vi "Calculate Response.vi"(0 "Neural Network In":T1={"Weigths"=[], "Last Layer Linear"=TRUE, "Add Bias Inputs"=TRUE, "# Inputs"=0, "# Output Neurons/Outputs"=0, "Inputs Scaling"={"X Scaling Vector"=[], "Y Scaling Vector"=[]}, "Outputs Scaling"={"X Scaling Vector"=[], "Y Scaling Vector"=[]}}, 5 "Inputs":dbl[](array[numeric]), 11 "Error In":errorcluster) -> (4 "Neural Network Out":T1={"Weigths"=[], "Last Layer Linear"=TRUE, "Add Bias Inputs"=TRUE, "# Inputs"=0, "# Output Neurons/Outputs"=0, "Inputs Scaling"={"X Scaling Vector"=[], "Y Scaling Vector"=[]}, "Outputs Scaling"={"X Scaling Vector"=[], "Y Scaling Vector"=[]}}, 6 "Outputs":dbl[](array[numeric]), 15 "Error Out":errorcluster)   [LabVIEW 2013, in "Super Simple Neural Network.lvlib"]
doc: "This VI calculates the output values of the network based on the input values. \n\nThis VI also uses the scaling information generated by the teaching algorithm to scale the inputs and outputs of the network. This means that you can work with any values as long as you have tought the network in that specific range."
uses:
  Super Simple Neural Network.lvlib
  Types/Neural Network.ctl
  Types/2D Array.ctl
  Types/Scaling Info.ctl
  <vilib>/Analysis/baseanly.llb/A x Vector.vi
  <vilib>/Analysis/NI_AALBase.lvlib
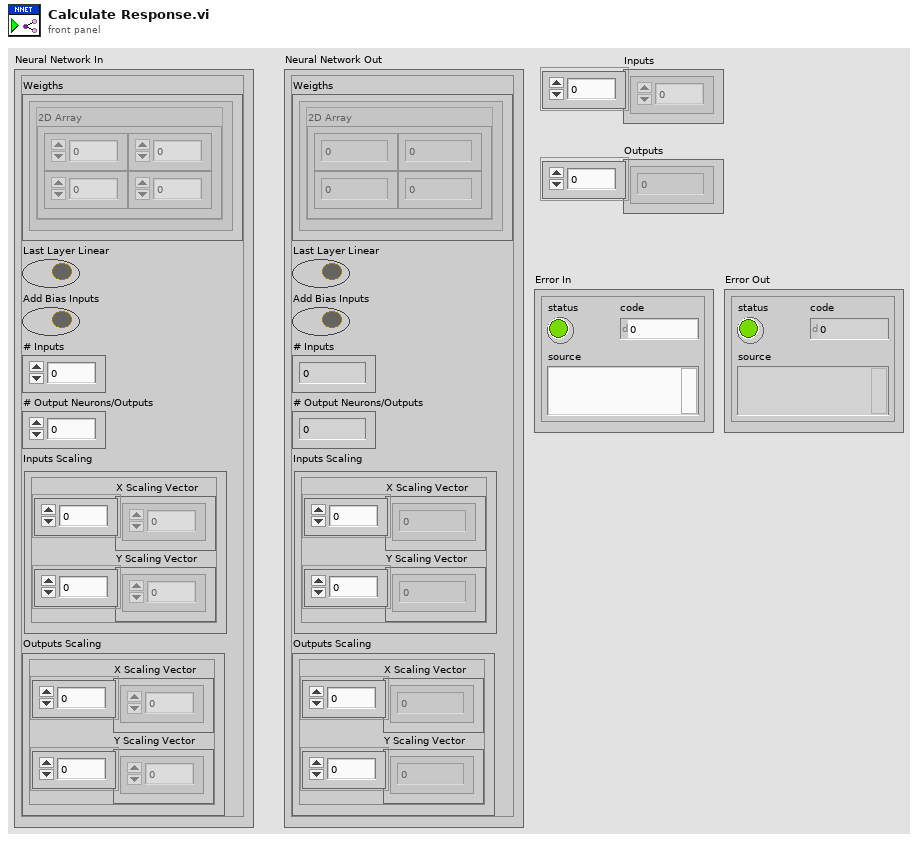
[diagram p1: front panel]
types:
  T1 = typedef "Super Simple Neural Network.lvlib/Neural Network.ctl" = cluster{"Weigths":T2[], "Last Layer Linear":bool, "Add Bias Inputs":bool, "# Inputs":u32, "# Output Neurons/Outputs":u32, "Inputs Scaling":T3, "Outputs Scaling":T3}
  T2 = typedef "Super Simple Neural Network.lvlib/2D Array.ctl" = cluster{"2D Array":dbl[][]}
  T3 = typedef "Super Simple Neural Network.lvlib/Scaling Info.ctl" = cluster{"X Scaling Vector":dbl[], "Y Scaling Vector":dbl[]}
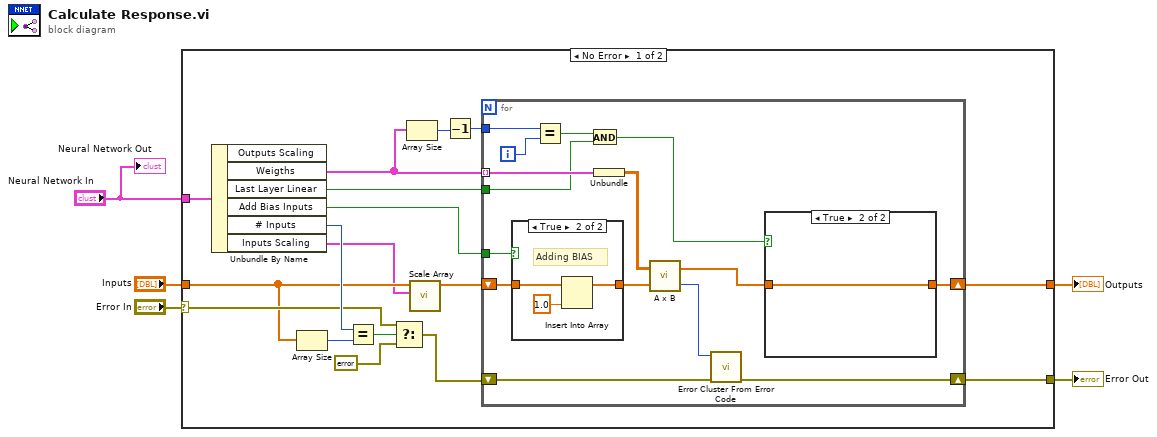
[diagram p0: block diagram]
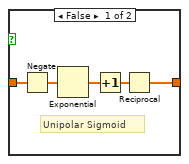
[diagram p3: hidden frame]
diagram:
  n1 = case shown="No Error" "Error In" {
    selector: "Error In" -> [w19 w48]
    tunnel: "Neural Network In" -> [w21 _]
    tunnel: "Inputs" -> [w15 _]
    tunnel: [w18 w48] -> w2
    tunnel: [w6 _] -> w1
    frame No Error {
      n2 = Unbundle By Name(w21) -> ("Weigths"=w17:T2[], "Last Layer Linear"=w16:bool, "Add Bias Inputs"=w22:bool, "# Inputs"=w20:u32, "Inputs Scaling"=w14:T3)  [unwired: 1 out]
      n3 = Array Size(array=w15) -> (size(s)=w10:i32)
      n4 = Equal?(x=w20, y=w10) -> (x = y?=w11:bool)
      n5 = Select(t=w19, s=w11, f=errorcluster {"status"=TRUE, "code"=5777, "source"="Number of inputs not equal to the expected number of inputs for this network."}) -> (s? t:f=w9:errorcluster)
      n6 = Array Size(array=w17) -> (size(s)=w13:i32)
      n7 = call "Scale Array.vi"("Scaling Info"=w14, "Array to Scale"=w15) -> ("Scaled Array"=w7:dbl[])  [unwired: 9 in]
      n8 = Decrement(x=w13) -> (x-1=w12:i32)
      n9 = for {
        shift-right: [w35] -> w6
        shift-left: w7 -> [w34]
        tunnel: w17 -> [w37] mode=indexing
        tunnel: w12 -> [w31]
        tunnel: w22 -> [w29]
        shift-right: [w25] -> w18
        shift-left: w9 -> [w26]
        tunnel: w16 -> [w23]
        i -> [w28]
        n10 = case shown="True" w29 {
          tunnel: w34 -> [w38 w40]
          tunnel: [w38 w39] -> w33
          frame False {
          }
          frame True {
            # "Adding BIAS"
            n11 = Insert Into Array(array=w40, new element=1.0 ("new element/subarray")) -> (w39:dbl[])  [unwired: 1 in]
          }
        }
        n12 = Equal?(x=w31, y=w28) -> (x = y?=w30:bool)
        n13 = And(x=w30, y=w23) -> (x .and. y?=w24:bool)
        n14 = Unbundle(w37) -> ("2D Array"=w36:dbl[][])
        n15 = call-poly <vilib>:"A x B.vi"("Vector"=w33, "A"=w36) -> ("error"=w27:i32, "A x Vector"=w32:dbl[])
        n16 = call <vilib>:"Error Cluster From Error Code.vi"("error in (no error)"=w26, "error code (0)"=w27) -> ("error out"=w25:errorcluster)  [unwired: 7 in]
        n17 = case shown="True" w24 {
          tunnel: [w43 w47] -> w35
          tunnel: w32 -> [w42 w47]
          frame False {
            # "Unipolar Sigmoid"
            n18 = Negate(x=w42) -> (-x=w46:dbl[])
            n19 = Exponential(1:w46) -> (0:w45:dbl[])
            n20 = Increment(x=w45) -> (x+1=w44:dbl[])
            n21 = Reciprocal(x=w44) -> (1/x=w43:dbl[])
          }
          frame True {
          }
        }
      }
    }
    frame Error {
    }
  }
  "Error Out" <- w2
  "Outputs" <- w1
  "Neural Network Out" <- "Neural Network In"
